vi "Read Output.vi"(8 "error in (no error)":errorcluster, 11 "VISA resource name":refnum<visa-resource-name>) -> (0 "error out":errorcluster, 1 "Displayed Current Value":dbl format="%.1g", 2 "Displayed Voltage Value":dbl format="%.2g", 3 "VISA resource name out":refnum<visa-resource-name>, 4 "CC/CV model":bool)   [LabVIEW 2022 SP3, in "BK Precision 9103.lvlib"]
doc: "Returns the actual voltage level and actual current level for a desired channel."
uses:
  <instrlib>/BK Precision 9103/BK Precision 9103.lvlib
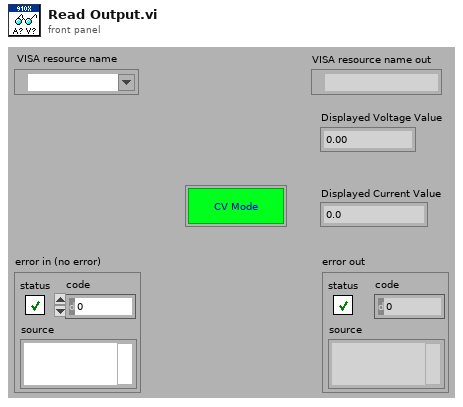
[diagram p1: front panel]
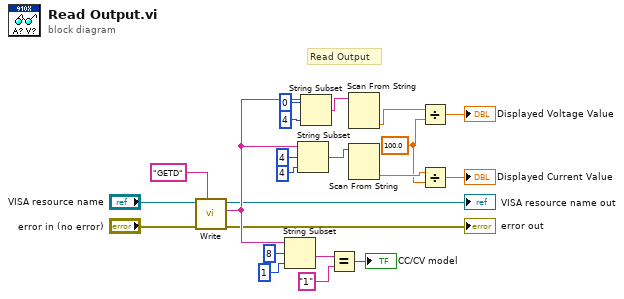
[diagram p0: block diagram]
diagram:
  w13 = 100.0 ("y")
  # "Read Output"
  n1 = call <instrlib>:"Write.vi"("Input String"="GETD", "error in (no error)"="error in (no error)", "VISA resource name"="VISA resource name") -> ("error out"=→"error out":errorcluster, "String"=w3:string, "VISA resource name out"=→"VISA resource name out":refnum<visa-resource-name>)  [unwired: 6 in]
  n2 = String Subset(string=w3, offset (0)=8, length (rest)=1 ("length (rest)")) -> (substring=w8:string)
  n3 = String Subset(string=w3, offset (0)=4, length (rest)=4 ("length (rest)")) -> (substring=w20:string)
  n4 = String Subset(string=w3, offset (0)=0, length (rest)=4 ("length (rest)")) -> (substring=w21:string)
  n5 = Equal?(x=w8, y="1" ("substring")) -> (x = y?=→"CC/CV model":bool)
  n6 = Scan From String(input string=w21) -> (output 1=w17:dbl)  [unwired: 4 in, 3 out]
  n7 = Scan From String(input string=w20) -> (output 1=w16:dbl)  [unwired: 4 in, 3 out]
  n8 = Divide(x=w17, y=w13) -> (x/y=→"Displayed Voltage Value":dbl)
  n9 = Divide(x=w16, y=w13) -> (x/y=→"Displayed Current Value":dbl)
